vi "list peak vs energy.vi"(11 "List":string[][](array[string])) -> (3 "List Peaks vs. Energy":string[][](table))   [LabVIEW 2020]
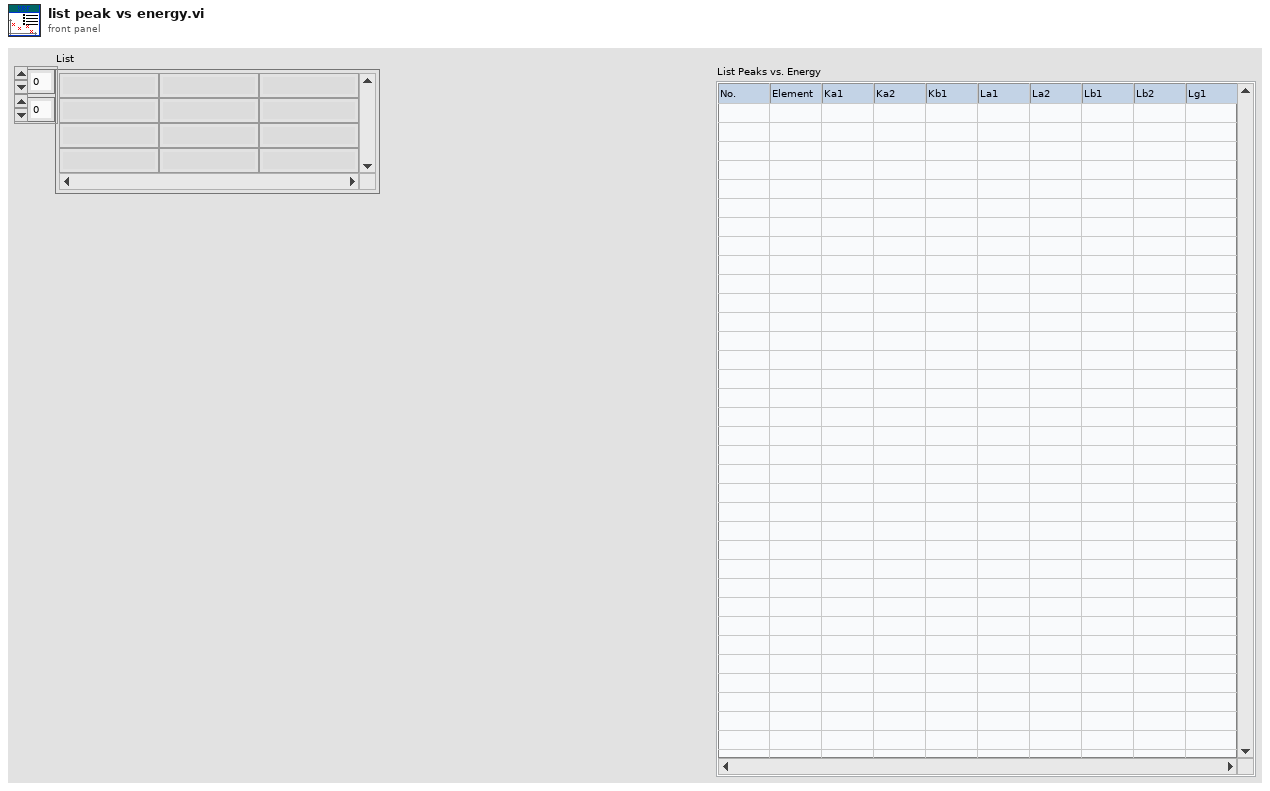
[diagram p1: front panel]
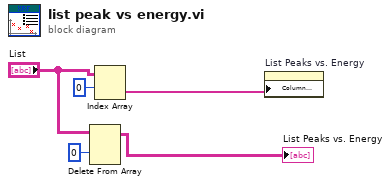
[diagram p0: block diagram]
diagram:
  n1 = Delete From Array(array="List", index (row)=0) -> (array with subset deleted=→"List Peaks vs. Energy":string[][])  [unwired: 2 in, 1 out]
  n2 = Index Array(array="List", index (row)=0) -> (element=w4:string[])  [unwired: 1 in]
  n3 = property on="List Peaks vs. Energy" class="Tbl (strict)"("Column Headers[]"=w4) -> ()  [unwired: 2 in, 2 out]
